vi "I32 to Matlab String.vi"(8 "error in (no error)":errorcluster, 10 "Value":i32, 11 "Variable name":string) -> (0 "error out":errorcluster, 3 "String":string)   [LabVIEW 2014, in "Matlab API.lvlib"]
uses:
  Matlab API.lvlib
panel:
  out "Array":u8[](array[numeric]) format="%x"
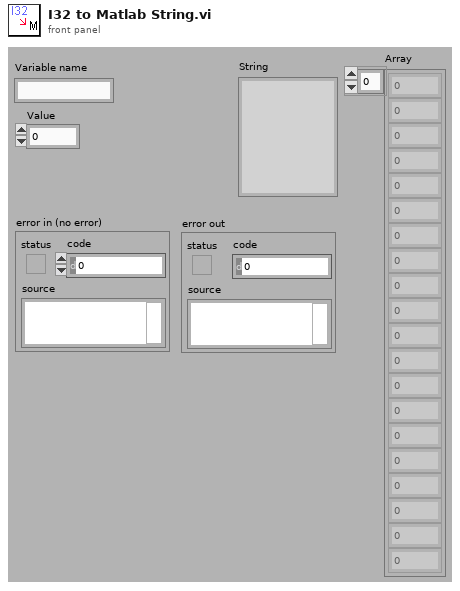
[diagram p1: front panel]
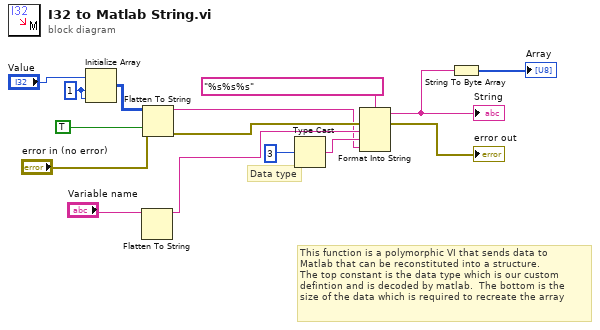
[diagram p0: block diagram]
diagram:
  w2 = 1 ("dimension size")
  # "Data type"
  # "This function is a polymorphic VI that sends data to\nMatlab that can be reconstituted into a structure.\nThe top constant is the data type which is our custom\ndefintion and is decoded by matlab.  The bottom is the\nsize of the data which is required to recreate the array"
  n1 = Initialize Array("Value", w2, w2) -> (w1:i32[][])
  n2 = Flatten To String(anything="Variable name") -> (data string=w5:string)  [unwired: 1 in, 4 out]
  n3 = Flatten To String(anything=w1, prepend array or string size? (T)=TRUE, error in (no error)="error in (no error)") -> (data string=w4:string, error out=w12:errorcluster)  [unwired: 2 out]
  n4 = Type Cast(x=3 ("input 2")) -> (*(type *) &x=w9:string)  [unwired: 1 out]
  n5 = Format Into String(format string="%s%s%s", error in=w12, w5, w9, w4) -> (resulting string=w7:string, error out=→"error out":errorcluster)  [unwired: 1 in]
  "String" <- w7
  n6 = String To Byte Array(string=w7) -> (unsigned byte array=→"Array":u8[])
